vi "uploadJudge.vi"(9 "passYield":dbl, 10 "pn":string, 11 "DBSet":T1) -> (3 "upload":bool)   [LabVIEW 2011]
panel:
  out "结果字符串":string
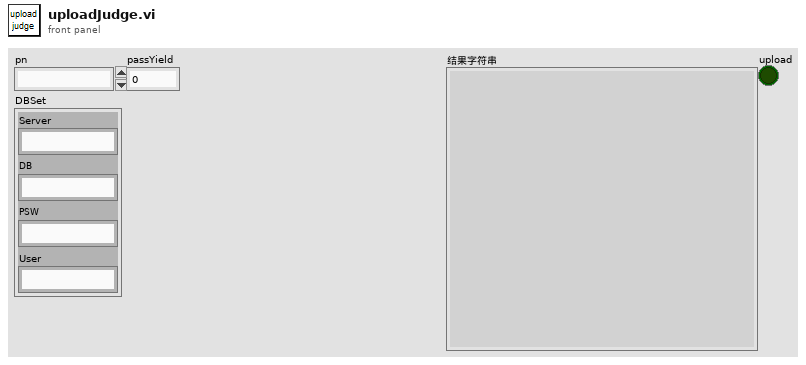
[diagram p1: front panel]
types:
  T1 = cluster{"Server":string, "DB":string, "PSW":string, "User":string}
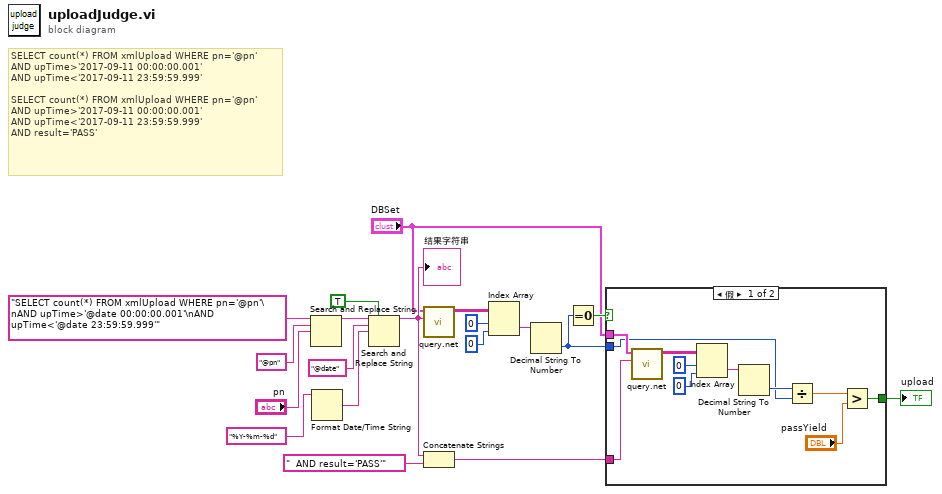
[diagram p0: block diagram]
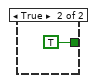
[diagram p2: hidden frame]
diagram:
  # "SELECT count(*) FROM xmlUpload WHERE pn='@pn'\nAND upTime>'2017-09-11 00:00:00.001'\nAND upTime<'2017-09-11 23:59:59.999'\n\nSELECT count(*) FROM xmlUpload WHERE pn='@pn'\nAND upTime>'2017-09-11 00:00:00.001'\nAND upTime<'2017-09-11 23:59:59.999'\nAND result='PASS'"
  n1 = Search and Replace String(input string="SELECT count(*) FROM xmlUpload WHERE pn='@pn'\nAND upTime>'@date 00:00:00.001'\nAND upTime<'@date 23:59:59.999'", search string="@pn" ("搜索字符串"), replace string="pn") -> (result string=w16:string)  [unwired: 5 in, 3 out]
  n2 = Format Date/Time String(time format string (%c)="%Y-%m-%d" ("时间格式字符串(%c)")) -> (date/time string=w14:string)  [unwired: 2 in]
  n3 = Search and Replace String(replace all?=TRUE ("替换全部？(F)"), input string=w16, search string="@date" ("搜索字符串"), replace string=w14) -> (result string=w10:string)  [unwired: 4 in, 3 out]
  "结果字符串" <- w10
  n4 = call "query.net.vi"("Sql"=w10, "DBSet"="DBSet") -> ("result"=w9:string[][])  [unwired: 8 in, 1 out]
  n5 = Concatenate Strings(w10, "  AND result='PASS'" ("字符串")) -> (w3:string)
  n6 = Index Array(array=w9, index (row)=0 ("索引 (行)"), index (col)=0 ("禁用的索引 (列)")) -> (element=w6:string)
  n7 = Decimal String To Number(string=w6) -> (number=w2:i32)  [unwired: 2 in, 1 out]
  n8 = Equal To 0?(x=w2) -> (x = 0?=w5:bool)
  n9 = case shown="假" w5 {
    tunnel: [w20 TRUE] -> w1
    tunnel: "DBSet" -> [w30 _]
    tunnel: w3 -> [w29 _]
    tunnel: w2 -> [w23 _]
    frame False {
      n10 = call "query.net.vi"("Sql"=w29, "DBSet"=w30) -> ("result"=w28:string[][])  [unwired: 8 in, 1 out]
      n11 = Index Array(array=w28, index (row)=0 ("索引 (行)"), index (col)=0 ("禁用的索引 (列)")) -> (element=w25:string)
      n12 = Decimal String To Number(string=w25) -> (number=w24:i32)  [unwired: 2 in, 1 out]
      n13 = Divide(x=w24, y=w23) -> (x/y=w22:dbl)
      n14 = Greater?(x=w22, y="passYield") -> (0:w20:bool)
    }
    frame True {
    }
  }
  "upload" <- w1
